vi "add PID to configuration.vi"(8 "error in":errorcluster, 9 "index":i32, 10 "PID Element in":T1, 11 "Tagbus PID Module configuration in":refnum<class "PID Module configuration.lvclass">) -> (0 "error out":errorcluster, 3 "Tagbus PID Module configuration out":refnum<class "PID Module configuration.lvclass">)   [LabVIEW 2015, in "PID Module configuration.lvclass"]
doc: "This VI takes in a PID Loop configuration, verifies that it's not currently in the Module Configuration object, and adds it to the Module Configuration at the specified index."
uses:
  PID Module configuration.lvclass
  editor node/PID array element.ctl
  PID Module configuration.lvclass/PID Module configuration.ctl
  PID Loop.lvclass
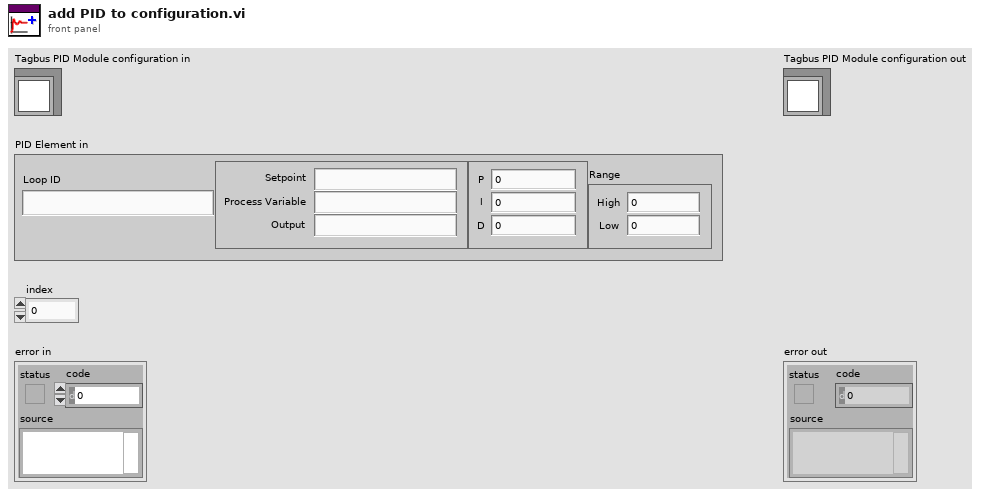
[diagram p1: front panel]
types:
  T1 = typedef "PID Module configuration.lvclass/PID array element.ctl" = cluster{"Loop ID":string, "Tags":cluster{"Setpoint":string, "Process Variable":string, "Output":string}, "Gains":cluster{"P":dbl, "I":dbl, "D":dbl}, "Range":cluster{"High":dbl, "Low":dbl}}
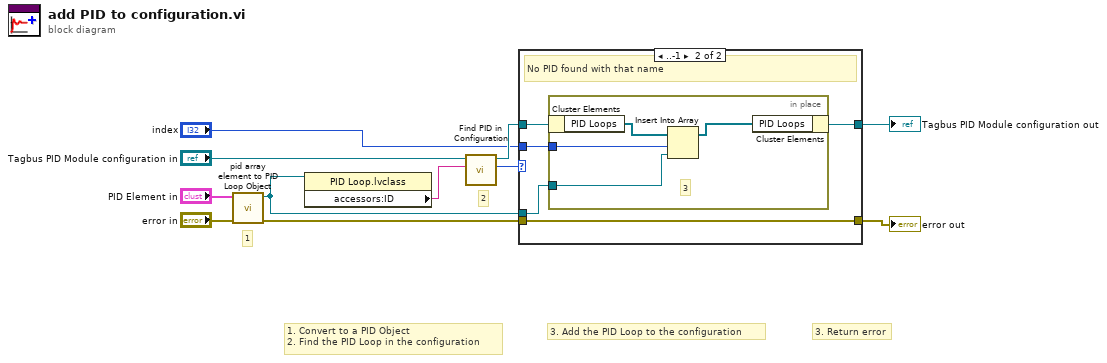
[diagram p0: block diagram]
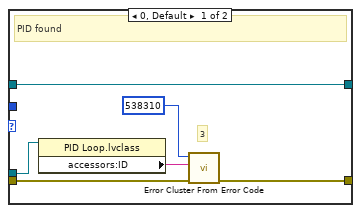
[diagram p2: hidden frame]
diagram:
  # "3. Return error"
  # "3. Add the PID Loop to the configuration"
  # "2"
  # "1. Convert to a PID Object\n2. Find the PID Loop in the configuration"
  # "1"
  n1 = call "pid array element to PID Loop Object.vi"("error in (no error)"="error in", "PID Element in"="PID Element in") -> ("error out"=w7:errorcluster, "PID Loop out"=w2:refnum<class "PID Loop.lvclass">)  [unwired: 8 in]
  n2 = property class="PID Loop.lvclass"(reference=w2) -> ("accessors:ID"=w3:string)  [unwired: 1 in, 2 out]
  n3 = call "Find PID in Configuration.vi"("PID Loop ID in"=w3, "Tagbus PID Module configuration in"="Tagbus PID Module configuration in") -> ("index"=w10:i32, "Tagbus PID Module configuration out"=w9:refnum<class "PID Module configuration.lvclass">)  [unwired: 8 in]
  n4 = case shown="..-1" w10 {
    tunnel: w9 -> [w14 w22]
    tunnel: w2 -> [w13 w19]
    tunnel: [w14 w21] -> w8
    tunnel: w7 -> [w16 w20]
    tunnel: [w15 w20] -> w6
    tunnel: "index" -> [_ w18]
    frame 0, Default {
      # "3"
      # "PID found"
      n5 = property class="PID Loop.lvclass"(reference=w13) -> ("accessors:ID"=w12:string)  [unwired: 1 in, 2 out]
      n6 = call <vilib>:"Error Cluster From Error Code.vi"("error in (no error)"=w16, "error message (\"\")"=w12, "error code (0)"=538310) -> ("error out"=w15:errorcluster)  [unwired: 6 in]
    }
    frame ..-1 {
      # "No PID found with that name"
      n7 = in-place {
        in-place-border: w19 -> [w24]
        in-place-border: w18 -> [w23]
        # "3"
        n8 = in-place-cluster #1(w22) -> ("PID Loops"=w26:refnum<class "PID Loop.lvclass">[])
        n9 = Insert Into Array(array=w26, index=w23, new element=w24) -> (w25:refnum<class "PID Loop.lvclass">[])
        n10 = in-place-cluster #1("PID Loops"=w25) -> (w21:refnum<class "PID Module configuration.lvclass">)
      }
    }
  }
  "error out" <- w6
  "Tagbus PID Module configuration out" <- w8
